vi "CPP_Aeroprobe.vi"() -> (5 "Plug in titles":string[](array[string]), 7 "Plug in values":string[](array[string]))   [LabVIEW 2022 SP3]
uses:
  Controls/AeroprobeType.ctl
  Controls/AeroprobeOrientation.ctl
  Plug in sub vis/CPP_Aeroprobe/eulerAngles.ctl
  <vilib>/Analysis/baseanly.llb/Mean (DBL).vi
  Globals/Meas_global.vi
  Globals/Constants_global.vi
  <vilib>/Utility/file.llb/Write Delimited Spreadsheet (DBL).vi
  <vilib>/Analysis/NI_AALBase.lvlib
panel:
  in  "manualOverride":bool
  in  "suppressNoiseWarning":bool
  out "PSU Warning":string
  in  "Probe:Euler:Angles":T1={"Roll"=-90.0, "Dip"=30.0, "Yaw"=0.0}
  out "Av Sampling Rate":dbl
  in  "Omniprobe Orientation":T2="30dip-EdgeTx {-90,30,0}"
  in  "Probe Type":T3=12 items=["5-Hole Probe"=5, "OmniProbe"=12]
  out "AeroFlow Output":cluster{string, string}[](array[cluster]) caption="Plug In Titles                                   Plug In Values"
  out "ZeroMeans&Vars":dbl[](array[numeric])
  in  "SaveTimeSeries?":bool
  in  "Mode":enum32{"Measure", "Take Zeroes"}(radio)
  in  "RunManually?":bool
  in  "MeanOrFull":bool
  in  "Graphs":bool
  in  "Downsampler":i32=40
  in  "Calibration Folder Path":path
  in  "Correction File Path":path
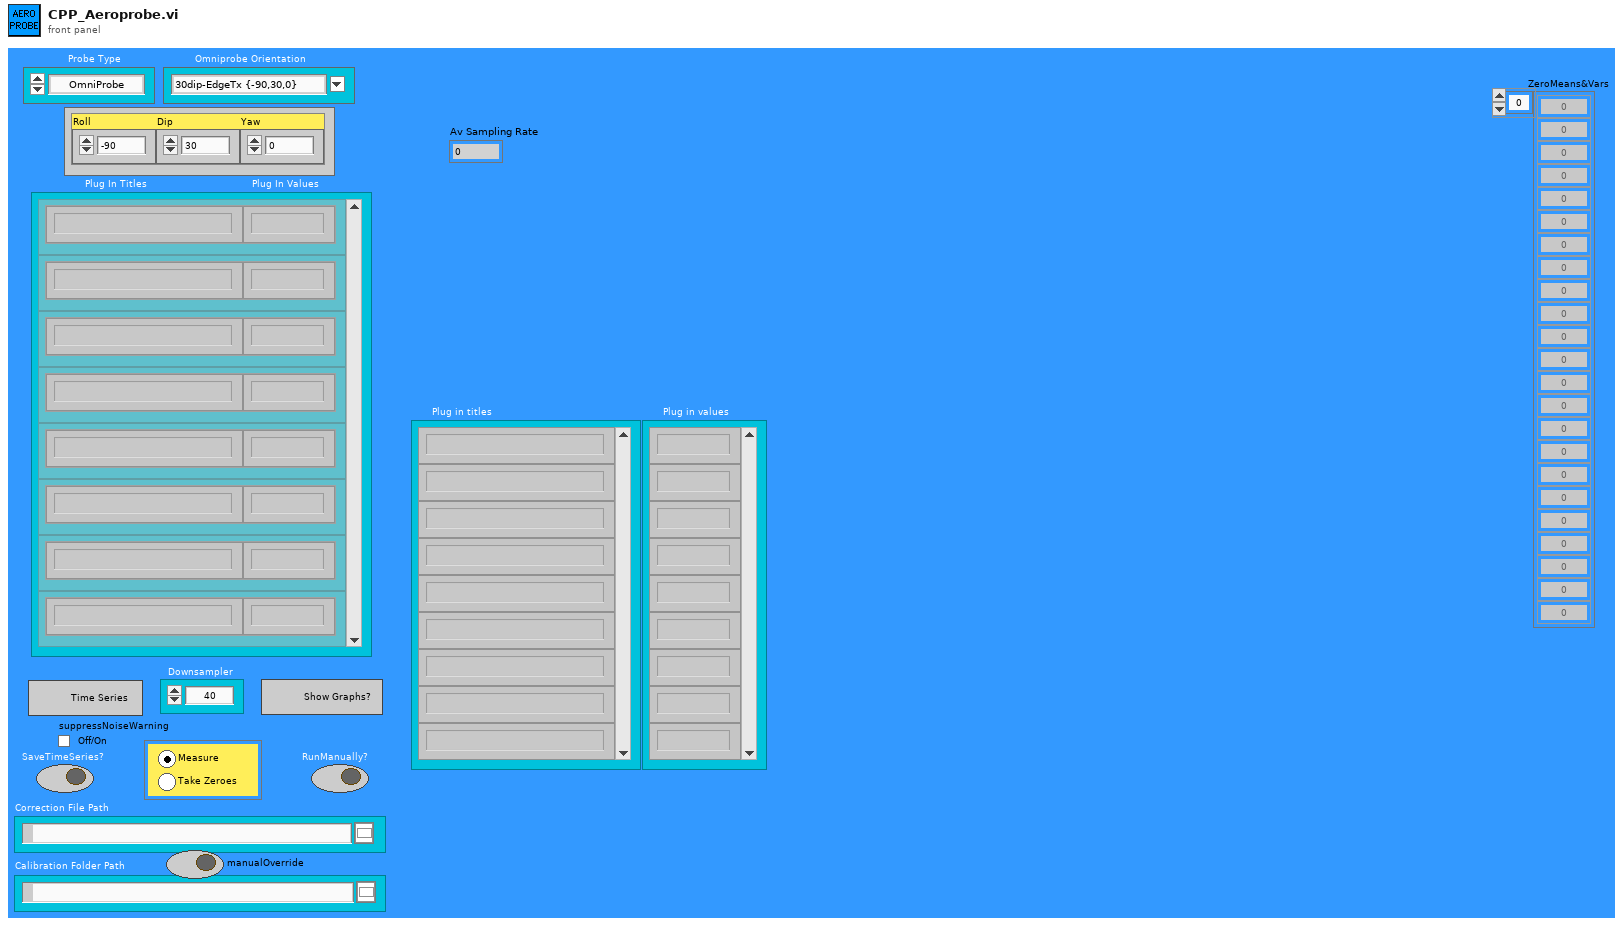
[diagram p1: front panel]
types:
  T1 = typedef "eulerAngles.ctl" = cluster{"Roll":dbl, "Dip":dbl, "Yaw":dbl}
  T2 = typedef "AeroprobeOrientation.ctl" = string
  T3 = typedef "AeroprobeType.ctl" = u16
  T4 = typedef "Post_Process.ctl" = enum16{"Take New Data", "Post Process Raw Data File"}
  T5 = enum16{"Raw Ends", "Mean Ends", "NaNd Ends", "Zeroed Ends"}
  T6 = enum16{"Save no data", "Save data in new files", "Save data in existing files"}
  T7 = typedef "Analysis_info_cluster.ctl" = cluster{"Colour":u32, "Inst type":T8, "Inst name":string, "Symbol":string, "Code name":string, "Extra Info":string, "Inst Array":T9, "Extra Titles":string[], "Extra Values":string[], "U":dbl, "u^2":dbl, "u^3":dbl, "u^4":dbl, "Skew_u":dbl, "Kurt_u":dbl, "Sd Error in Mean":dbl, "% u'/U":dbl, "X":dbl, "Y":dbl, "Z":dbl, "Timescale integral Estimate":dbl, "Sd Error in Variance":dbl, "Calib File":path, "Calib Constants":dbl[], "Output Position":bool, "Stats":enum16{"None", "Basic", "Full"}, "Av Sampling Rate":dbl, "Av No of Samples":dbl, "Total Meas Time (s)":dbl, "ADAM Ch Name":string, "Max value":dbl, "Min value":dbl, "Req Sample Rate Hz":dbl, "Sync Delay Time (s)":dbl, "Ch No":i16, "Device":string, "Use Latest Calib":bool, "Port":string, "Metadata Ch Names":string[], "Metadata Ch Values":string[], "Label":string}
  T8 = typedef "Inst_type.ctl" = enum16{"Raw voltage", "Raw with zero offsetting", "Propeller anemometer", "Pressure Transducer", "Pitot-static tube", "Hot wire", "Cross wire 1", "Cross wire 2", "Generic Linear", "Generic Polynomial", "Generic BackPoly", "Fast FID", "Thermocouple", "Cold wire", "Pulsed Wire", "LDA Vel", "LDA Tran time", "LDA Arr time", "Microphone"}
  T9 = typedef "Instrument_Array.ctl" = enum16{"PWA", "LDA", "Analogue"}
  T10 = typedef "Time_Trace_Cluster.ctl" = cluster{"Weighting":dbl[], "Voltage":dbl[], "Eng Values":dbl[]}
  T11 = cluster{"CleanVmagUVWCone":dbl[][], "CleanXvals":i32[]}
  T12 = typedef "SanityCluster.ctl" = cluster{"PressureErrors":bool[][], "Plug in titles":string[]}
  T13 = cluster{"   Vmag          U               V              W        Cone":dbl[][], "Xvals":i32[]}
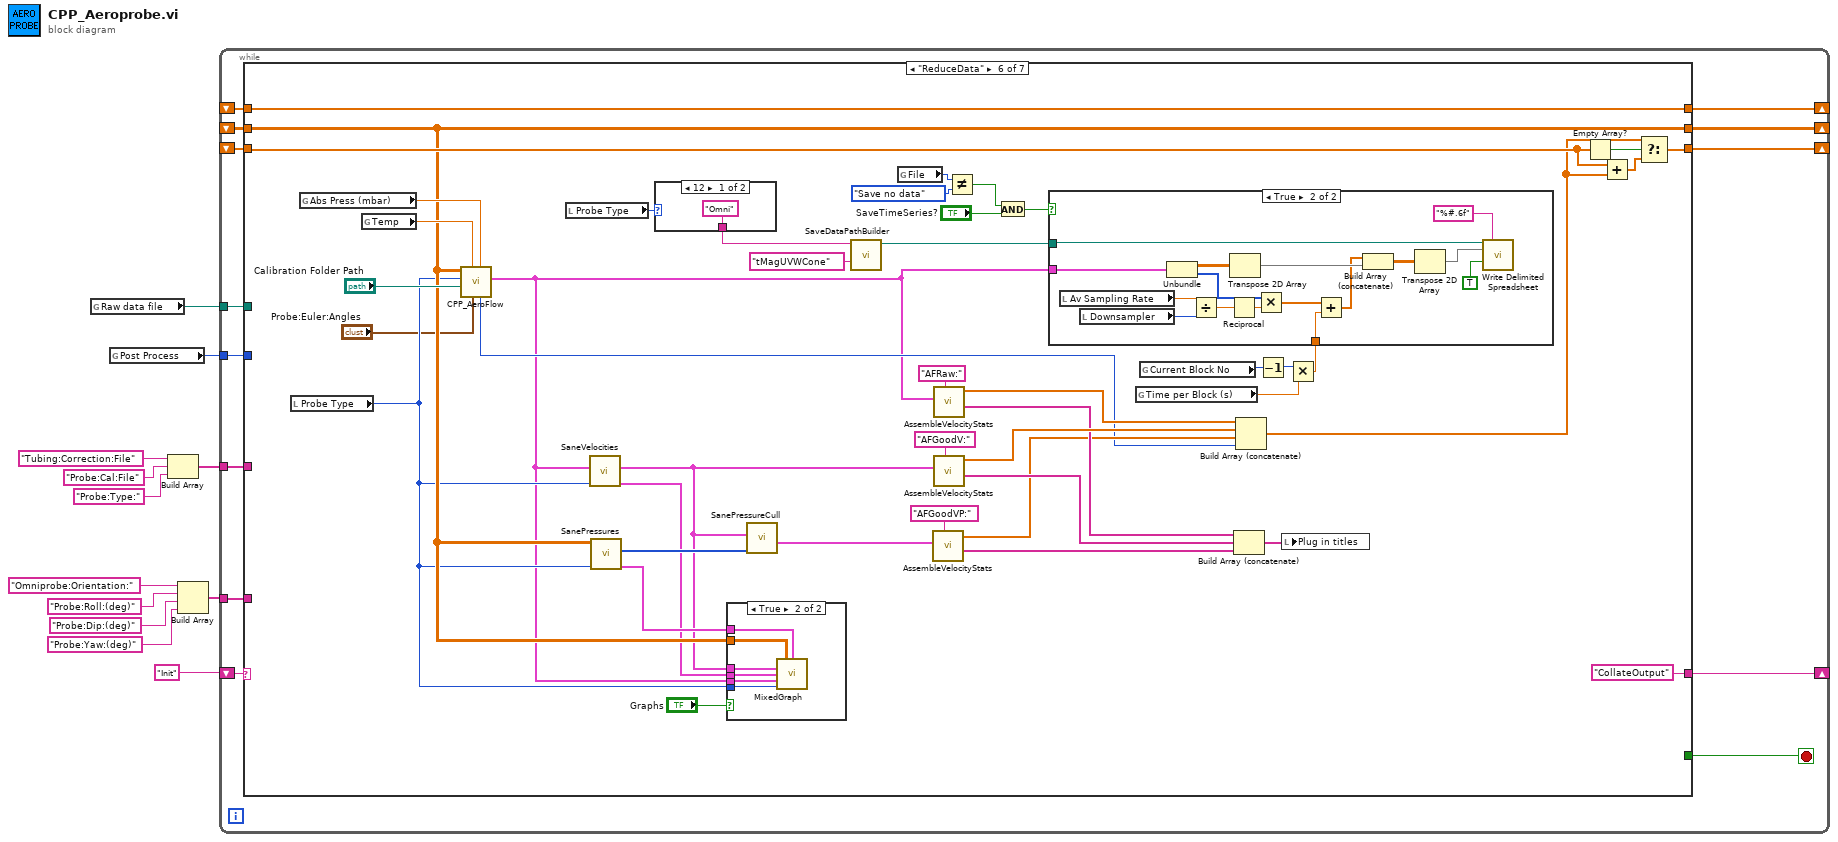
[diagram p0: block diagram]
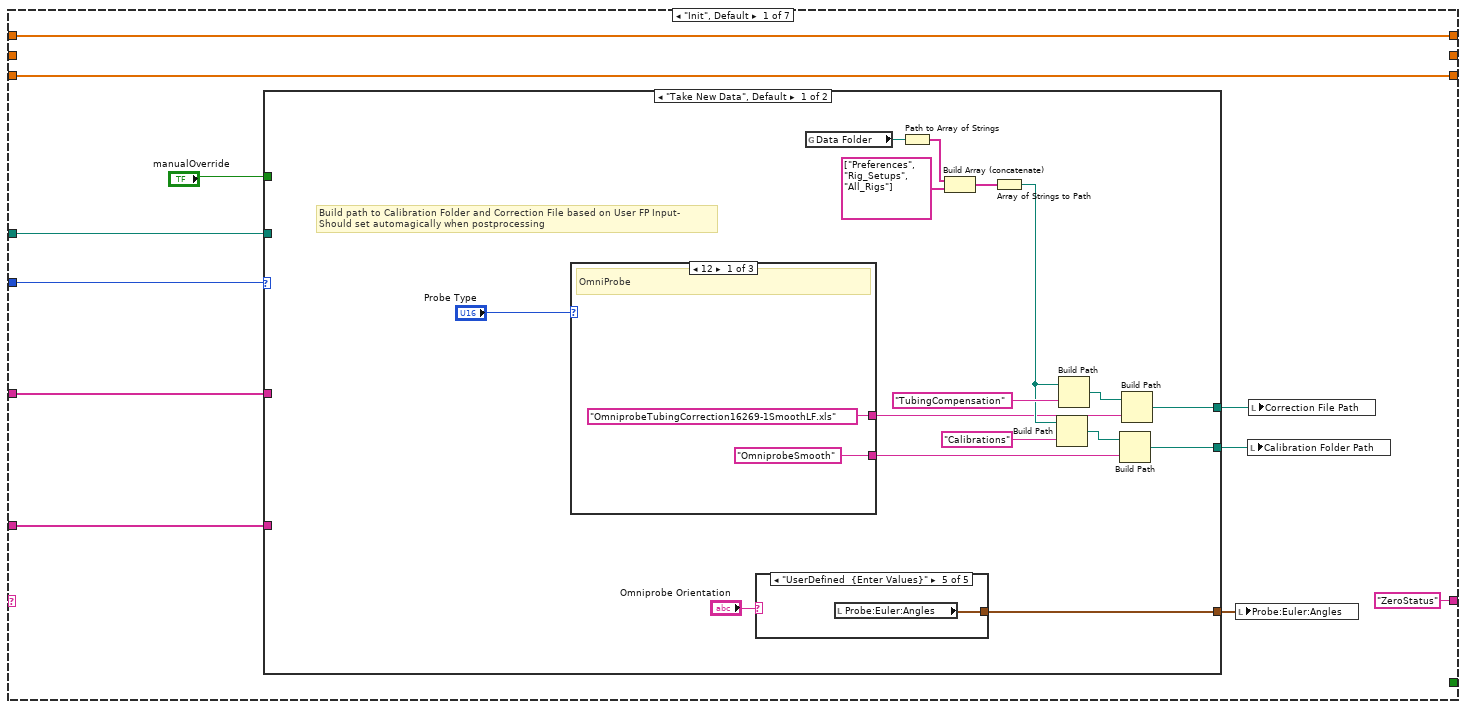
[diagram p2: hidden frame]
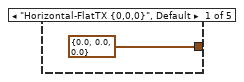
[diagram p3: hidden frame]
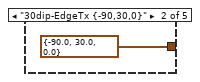
[diagram p4: hidden frame]
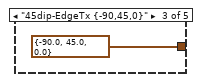
[diagram p5: hidden frame]
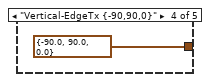
[diagram p6: hidden frame]
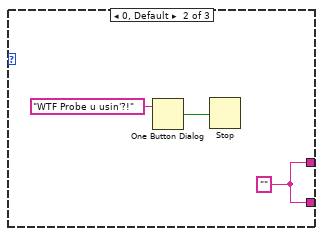
[diagram p7: hidden frame]
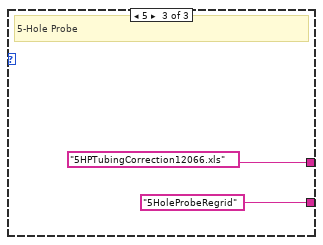
[diagram p8: hidden frame]
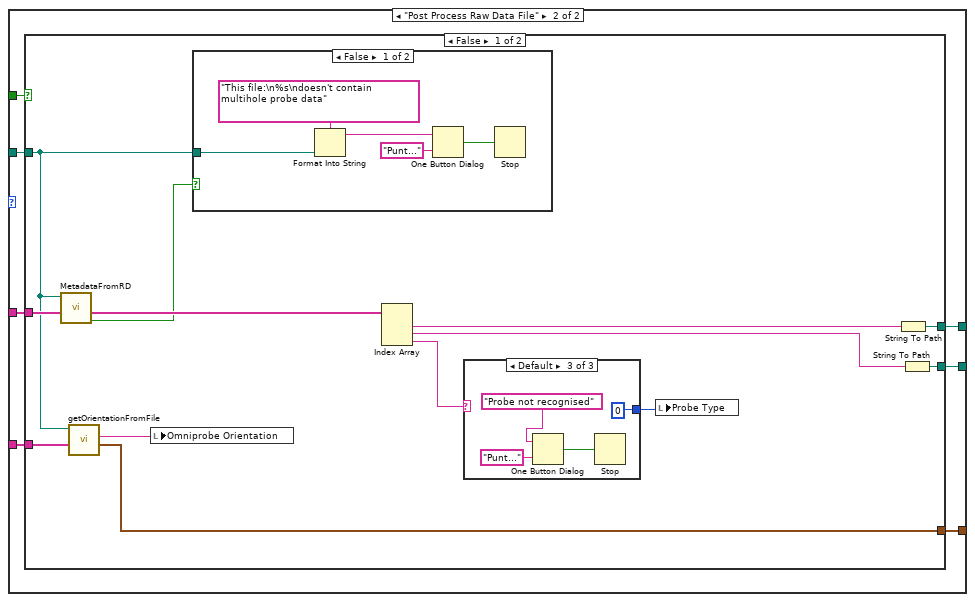
[diagram p9: hidden frame]
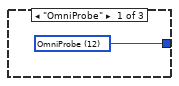
[diagram p10: hidden frame]
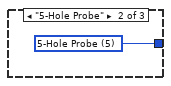
[diagram p11: hidden frame]
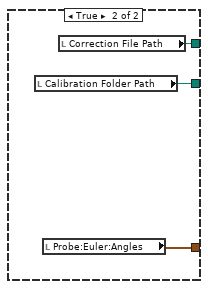
[diagram p13: hidden frame]
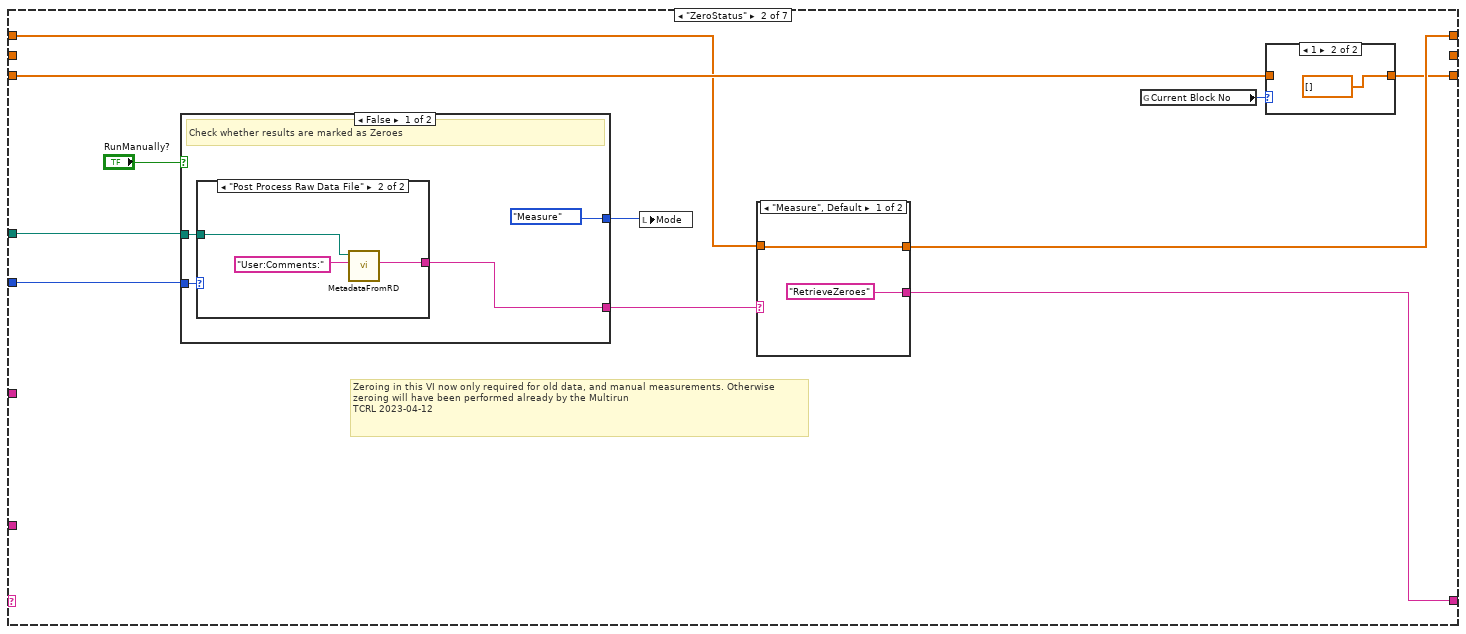
[diagram p14: hidden frame]
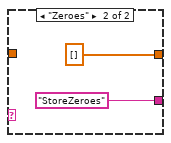
[diagram p15: hidden frame]
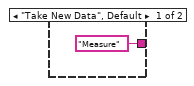
[diagram p16: hidden frame]
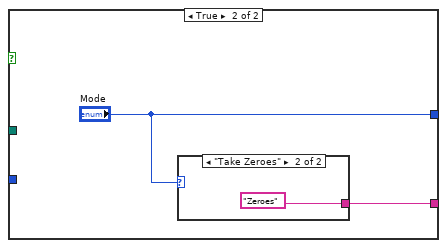
[diagram p17: hidden frame]
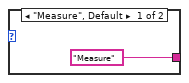
[diagram p18: hidden frame]
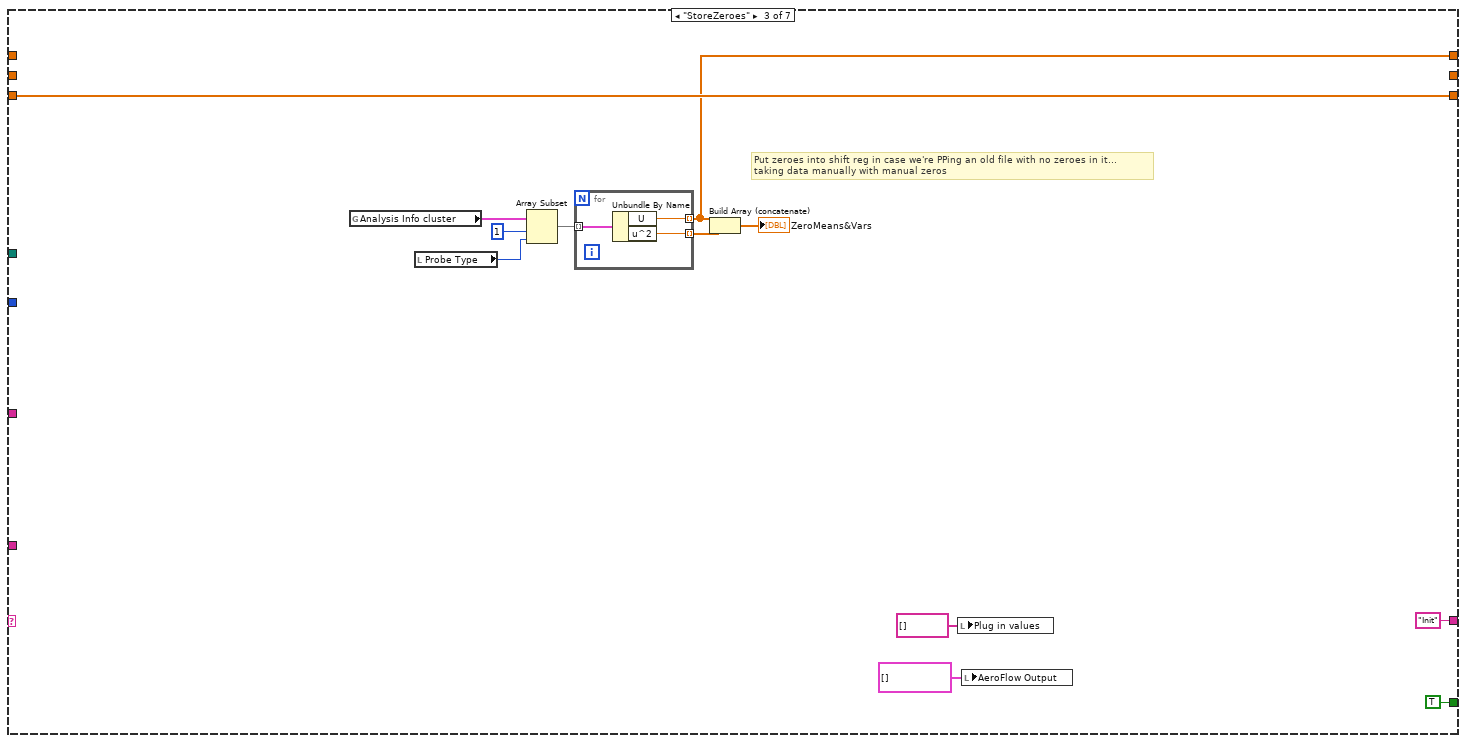
[diagram p20: hidden frame]
diagram:
  n1 = global read "Meas_global.vi" "Raw data file"() -> (w1:path)
  n2 = global read "Meas_global.vi" "Post Process"() -> (w11:T4)
  n3 = Build Array("Tubing:Correction:File" ("element"), "Probe:Cal:File" ("element"), "Probe:Type:" ("element")) -> (w4:string[])
  n4 = Build Array("Omniprobe:Orientation:" ("element"), "Probe:Roll:(deg)" ("element"), "Probe:Dip:(deg)" ("element"), "Probe:Yaw:(deg)" ("element")) -> (w6:string[])
  n5 = while {
    shift-right: [w24] -> _
    shift-left: "Init" -> [w25]
    shift-right: [w23] -> _
    shift-left: _ -> [w22]
    shift-right: [w21] -> _
    shift-left: _ -> [w20]
    shift-right: [w18] -> _
    shift-left: _ -> [w17]
    tunnel: w11 -> [w16]
    tunnel: w6 -> [w15]
    tunnel: w4 -> [w14]
    tunnel: w1 -> [w13]
    stop <- w19 stop-if-true
    n6 = case shown="\"ReduceData\"" w25 {
      tunnel: ["ZeroStatus" w101 "Init" w152 "ReduceData" "CollateOutput" "Init"] -> w24
      tunnel: [w36 w109 w133 w147 w191 w286 w348] -> w23
      tunnel: w22 -> [w36 w102 _ w149 w191 w286 w348]
      tunnel: [w35 w108 w139 w155 w193 w282 w342] -> w21
      tunnel: w20 -> [w35 w107 w139 w155 w193 w285 w342]
      tunnel: [_ _ TRUE w151 FALSE _ TRUE] -> w19
      tunnel: [_ _ _ w154 w188 w258 w344] -> w18
      tunnel: w17 -> [_ _ _ w154 _ w258 w344]
      tunnel: w16 -> [w31 w100 _ _ _ _ _]
      tunnel: w15 -> [w28 _ _ _ _ _ w314]
      tunnel: w14 -> [w30 _ _ _ _ _ w312]
      tunnel: w13 -> [w29 w99 _ w143 _ _ _]
      frame "Init", Default {
        n7 = case shown="\"Take New Data\", Default" w31 {
          tunnel: [w41 w69] -> w33
          tunnel: [w40 w70] -> w32
          tunnel: w30 -> [_ w71]
          tunnel: w29 -> [_ w68]
          tunnel: w28 -> [_ w67]
          tunnel: [w37 w66] -> w27
          tunnel: "manualOverride" -> [_ w65]
          frame "Take New Data", Default {
            # "Build path to Calibration Folder and Correction File based on User FP Input-\nShould set automagically when postprocessing"
            n8 = case shown="12" "Probe Type" {
              tunnel: ["OmniprobeTubingCorrection16269-1SmoothLF.xls" ("Tubing Compensation File") w62 "5HPTubingCorrection12066.xls" ("Tubing Compensation File")] -> w45
              tunnel: ["OmniprobeSmooth" ("Calibration Folder") w62 "5HoleProbeRegrid" ("Calibration Folder")] -> w44
              frame 12 {
                # "OmniProbe"
              }
              frame 0, Default {
                w62 = "" ("Calibration Folder")
                n9 = One Button Dialog(message="WTF Probe u usin'?!") -> (true=w60:bool)  [unwired: 1 in]
                n10 = Stop(stop? (T)=w60) -> ()
              }
              frame 5 {
                # "5-Hole Probe"
              }
            }
            n11 = case shown="\"UserDefined  {Enter Values}\"" "Omniprobe Orientation" {
              tunnel: [T1 {"Roll"=0.0, "Dip"=0.0, "Yaw"=0.0} ("Probe:Euler:Angles") T1 {"Roll"=-90.0, "Dip"=30.0, "Yaw"=0.0} ("Probe:Euler:Angles") T1 {"Roll"=-90.0, "Dip"=45.0, "Yaw"=0.0} ("Probe:Euler:Angles") T1 {"Roll"=-90.0, "Dip"=90.0, "Yaw"=0.0} ("Probe:Euler:Angles") w57] -> w37
              frame "Horizontal-FlatTX {0,0,0}", Default {
              }
              frame "30dip-EdgeTx {-90,30,0}" {
              }
              frame "45dip-EdgeTx {-90,45,0}" {
              }
              frame "Vertical-EdgeTx {-90,90,0}" {
              }
              frame "UserDefined  {Enter Values}" {
                n12 = local read "Probe:Euler:Angles"() -> (w57:T1)
              }
            }
            n13 = global read "Constants_global.vi" "Data Folder"() -> (w49:path)
            n14 = Path to Array of Strings(0:w49) -> (2:w52:string[])  [unwired: 1 out]
            n15 = Build Array (concatenate)(w52, string[] ["Preferences", "Rig_Setups", "All_Rigs"] ("array of strings 3")) -> (w50:string[])
            n16 = Array of Strings to Path(0:w50) -> (2:w46:path)  [unwired: 1 in]
            n17 = Build Path(base path=w46, name or relative path="Calibrations") -> (appended path=w42:path)
            n18 = Build Path(base path=w46, name or relative path="TubingCompensation") -> (appended path=w43:path)
            n19 = Build Path(base path=w42, name or relative path=w44) -> (appended path=w41:path)
            n20 = Build Path(base path=w43, name or relative path=w45) -> (appended path=w40:path)
          }
          frame "Post Process Raw Data File" {
            n21 = case shown="False" w65 {
              tunnel: w71 -> [w84 _]
              tunnel: [w81 w98] -> w70
              tunnel: [w79 w97] -> w69
              tunnel: w68 -> [w76 _]
              tunnel: w67 -> [w75 _]
              tunnel: [w74 w96] -> w66
              frame False {
                n22 = call "MetadataFromRD.vi"("ChannelNames"=w84, "Raw data file"=w76) -> ("allFound"=w78:bool, "ValueStrings"=w83:string[])  [unwired: 6 in, 2 out]
                n23 = call "getOrientationFromFile.vi"("currentChannels"=w75, "Raw data file"=w76) -> ("Probe:Euler:Angles"=w74:T1, "Omniprobe:Orientation"=w77:string)  [unwired: 8 in]
                n24 = local write "Omniprobe Orientation"(w77) -> ()
                n25 = case shown="False" w78 {
                  tunnel: w76 -> [w91 _]
                  frame False {
                    n26 = Format Into String(format string="This file:\n%s\ndoesn't contain multihole probe data" ("message"), w91) -> (resulting string=w94:string)  [unwired: 2 in, 1 out]
                    n27 = One Button Dialog(message=w94, button name ("OK")="Punt...") -> (true=w95:bool)
                    n28 = Stop(stop? (T)=w95) -> ()
                  }
                  frame True {
                  }
                }
                n29 = Index Array(array=w83) -> (element #1=w82:string, element #2=w80:string, element #3=w73:string)  [unwired: 3 in]
                n30 = case shown="Default" w73 {
                  tunnel: [w85 w86 0] -> w72
                  frame "OmniProbe" {
                    w85 = T3 12 items=["5-Hole Probe"=5, "OmniProbe"=12] ("Probe Type")
                  }
                  frame "5-Hole Probe" {
                    w86 = T3 5 items=["5-Hole Probe"=5, "OmniProbe"=12] ("Probe Type")
                  }
                  frame Default {
                    n31 = One Button Dialog(message="Probe not recognised", button name ("OK")="Punt...") -> (true=w89:bool)
                    n32 = Stop(stop? (T)=w89) -> ()
                  }
                }
                n33 = local write "Probe Type"(w72) -> ()
                n34 = String To Path(string=w82) -> (path=w81:path)
                n35 = String To Path(string=w80) -> (path=w79:path)
              }
              frame True {
                n36 = local read "Calibration Folder Path"() -> (w97:path)
                n37 = local read "Probe:Euler:Angles"() -> (w96:T1)
                n38 = local read "Correction File Path"() -> (w98:path)
              }
            }
          }
        }
        n39 = local write "Probe:Euler:Angles"(w27) -> ()
        n40 = local write "Calibration Folder Path"(w33) -> ()
        n41 = local write "Correction File Path"(w32) -> ()
      }
      frame "ZeroStatus" {
        # "Zeroing in this VI now only required for old data, and manual measurements. Otherwise zeroing will have been performed already by the Multirun\nTCRL 2023-04-12"
        n42 = case shown="False" "RunManually?" {
          tunnel: [enum32{"Measure", "Take Zeroes"}."Measure" ("Mode") "Mode"] -> w104
          tunnel: w100 -> [w117 _]
          tunnel: [w115 w122] -> w103
          tunnel: w99 -> [w114 _]
          frame False {
            # "Check whether results are marked as Zeroes"
            n43 = case shown="\"Post Process Raw Data File\"" w117 {
              tunnel: ["Measure" ("ValueString") w120] -> w115
              tunnel: w114 -> [_ w119]
              frame "Take New Data", Default {
              }
              frame "Post Process Raw Data File" {
                n44 = call "MetadataFromRD.vi"("ChannelName"="User:Comments:", "Raw data file"=w119) -> ("ValueString"=w120:string)  [unwired: 6 in, 3 out]
              }
            }
          }
          frame True {
            n45 = case shown="\"Take Zeroes\"" "Mode" {
              tunnel: ["Measure" ("y") "Zeroes" ("y")] -> w122
              frame "Measure", Default {
              }
              frame "Take Zeroes" {
              }
            }
          }
        }
        n46 = local write "Mode"(w104) -> ()
        n47 = case shown="\"Measure\", Default" w103 {
          tunnel: [w111 dbl[] [] ("t")] -> w109
          tunnel: w102 -> [w111 _]
          tunnel: ["RetrieveZeroes" "StoreZeroes"] -> w101
          frame "Measure", Default {
          }
          frame "Zeroes" {
          }
        }
        n48 = global read "Meas_global.vi" "Current Block No"() -> (w106:i32)
        n49 = case shown="1" w106 {
          tunnel: [w126 dbl[] [] ("t")] -> w108
          tunnel: w107 -> [w126 _]
          frame 0, Default {
          }
          frame 1 {
          }
        }
      }
      frame "StoreZeroes" {
        # "Put zeroes into shift reg in case we're PPing an old file with no zeroes in it...\ntaking data manually with manual zeros"
        n50 = global read "Meas_global.vi" "Analysis Info cluster"() -> (w137:T7[])
        n51 = local read "Probe Type"() -> (w135:T3)
        n52 = Array Subset(array=w137, index=1, length=w135) -> (w136:T7[])
        n53 = for {
          tunnel: w136 -> [w142] mode=indexing
          tunnel: [w141] -> w133 mode=indexing
          tunnel: [w140] -> w134 mode=indexing
          n54 = Unbundle By Name(w142) -> ("U"=w141:dbl, "u^2"=w140:dbl)
        }
        n55 = Build Array (concatenate)(w133, w134) -> (→"ZeroMeans&Vars":dbl[])
        n56 = local write "Plug in values"(string[] [] ("Plug in values")) -> ()
        n57 = local write "AeroFlow Output"(cluster{string, string}[] [] ("AeroFlow Output")) -> ()
      }
      frame "RetrieveZeroes" {
        # "Didn't find zeroes- hope they're in shift register"
        # "Found all the zeroes we need"
        # "Usual punt if we didn't get any zeroes\nNew data will either have been pre-zeroed by multirun, or manually zeroed in shift register\nIf we're postprocessing old data, zeros will be retrieved from RawDataFile"
        n58 = local read "Probe Type"() -> (w144:T3)
        n59 = call "findZerosInRD.vi"("Probe Type"=w144, "Raw data file"=w143) -> ("zerosChannels"=w145:string[])  [unwired: 9 in]
        n60 = call "RetrieveMetadataLiveOrPost.vi"("ChannelsToGet"=w145) -> ("ChannelValues"=w148:dbl[])  [unwired: 10 in]
        n61 = Add Array Elements(numeric array=w148) -> (sum=w153:dbl)
        n62 = Not A Number/Path/Refnum?(number/path/refnum=w153) -> (NaN/Path/Refnum?=w150:bool)
        n63 = Select(t=w149, s=w150, f=w148) -> (s? t:f=w147:dbl[])
        n64 = Empty Array?(array=w147) -> ()  [unwired: 1 out]
        n65 = case shown="False" FALSE {
          tunnel: ["CompensateData" "Init"] -> w152
          tunnel: [FALSE TRUE] -> w151
          frame False {
          }
          frame True {
            n66 = One Button Dialog(message="No zeroes. Try again.", button name ("OK")="OK") -> ()  [unwired: 1 out]
          }
        }
      }
      frame "CompensateData" {
        w186 = 1  # skip Pitot on Ch0
        # "Only subtract zeroes if there are some"
        # "Only complain if PSU in measurements"
        # "#Brittle\nTo cope with various Meas Setups"
        # "#FilthyHack"
        # "Using end-NaNd version of boosted data, to avoid the FFT' kicks that are frequently observed; hopefully AeroFlow can cope with NaNs..?!"
        n67 = global read "Meas_global.vi" "Analysis Info cluster"() -> (w169:T7[])
        n68 = local read "Probe Type"() -> (w179:T3)
        n69 = for {
          tunnel: w169 -> [w199] mode=indexing
          tunnel: [w198] -> w168
          tunnel: [w197] -> w167
          tunnel: [w194] -> w164
          tunnel: string[] ["Vsupply", "5V", "PSU"] -> [w196]
          stop <- w194 stop-if-true
          n70 = Unbundle By Name(w199) -> ("Inst name"=w195:string, "U"=w198:dbl, "u^2"=w197:dbl)
          n71 = for {
            tunnel: w196 -> [w203] mode=indexing
            tunnel: w195 -> [w201]
            tunnel: [w200] -> w194
            stop <- w200 stop-if-true
            n72 = Match Pattern(string=w201, regular expression=w203) -> (offset past match=w202:i32)  [unwired: 1 in, 3 out]
            n73 = Greater Or Equal To 0?(x=w202) -> (x >= 0?=w200:bool)
          }
        }
        n74 = global read "Meas_global.vi" "Time Trace"() -> (w180:T10[])
        n75 = case shown="12, Default" w179 {
          tunnel: [3e-07 ("y") 3.2e-07 ("y")] -> w177
          tunnel: [5e-08 ("y") 5e-08 ("y")] -> w178
          tunnel: [4.98 ("upper limit") 4.98 ("upper limit")] -> w176
          tunnel: [5.01 ("upper limit") 5.01 ("upper limit")] -> w175
          frame 5 {
          }
          frame 12, Default {
          }
        }
        n76 = Array Subset(array=w180, index=w186, length=w179) -> (w185:T10[])
        n77 = Index Array(array=w169, index=1) -> (element=w183:T7)
        n78 = Unbundle By Name(w183) -> ("Av Sampling Rate"=w181:dbl)
        "Av Sampling Rate" <- w181
        n79 = for {
          tunnel: w185 -> [w221] mode=indexing
          tunnel: [w220] -> w184 mode=indexing
          n80 = Unbundle By Name(w221) -> ("Eng Values"=w220:dbl[])
        }
        n81 = In Range and Coerce(upper limit=w175, x=w168, lower limit=w176) -> (In Range?=w174:bool)  [unwired: 1 out]
        n82 = In Range and Coerce(upper limit=w177, x=w167, lower limit=w178) -> (In Range?=w173:bool)  [unwired: 1 out]
        n83 = global read "Meas_global.vi" "Post Process"() -> (w172:T4)
        n84 = Compound Arithmetic op=OR(invert w174, invert w173) -> (w166:bool)
        n85 = Compound Arithmetic op=AND(w164, w166, invert "suppressNoiseWarning") -> (w165:bool)
        n86 = case shown="False" "MeanOrFull" {
          tunnel: [w226 w241] -> w192
          tunnel: w184 -> [w225 w240]
          tunnel: w181 -> [w222 _]
          frame False {
            # "Get the data off the global, and apply acoustic tubing correction. \nThen throw 90% of it away because we can't reduce it fast enough!"
            n87 = for {
              tunnel: w225 -> [w238] mode=indexing
              tunnel: [w235] -> w229 mode=indexing
              tunnel: TRUE ("Apply Phase Correction?") -> [w237]
              tunnel: "Correction File Path" -> [w236]
              tunnel: T5."NaNd Ends" ("EndTreatment") -> [w234]
              tunnel: 1.0 ("EndTrimLength(%)") -> [w233]
              tunnel: w222 -> [w232]
              workers-P: _ -> [_]
              n88 = call "GetCoeffsAndComp.vi"("EndTrimLength(%)"=w233, "EndTreatment"=w234, "Apply Phase Correction?"=w237, "Actual Sampling rate (Hz)"=w232, "mutedData"=w238, "TubingCorrectionFile"=w236) -> ("boostedData"=w235:dbl[])  [unwired: 5 in]
            }
            n89 = Transpose 2D Array(2D array=w229) -> (transposed array=w228:dbl[][])
            n90 = call "Decimator.vi"("Decimator"="Downsampler", "Array In"=w228) -> ("DecimatedArrayOut"=w226:dbl[][])  [unwired: 9 in]
          }
          frame True {
            # "Quick-and-dirty reduction of mean pressures"
            n91 = for {
              tunnel: w240 -> [w243] mode=indexing
              tunnel: [w242] -> w239 mode=indexing
              n92 = call-poly <vilib>:"Mean.vi"("X"=w243) -> ("mean"=w242:dbl)  [unwired: 1 out]
            }
            n93 = Build Array(w239) -> (w241:dbl[][])
          }
        }
        n94 = case shown="True" w165 {
          tunnel: w172 -> [_ w208]
          tunnel: ["" "Warning!\nAeroprobe PSU out of tolerance" ("PSU Warning")] -> w171
          tunnel: [FALSE ("Visible") TRUE ("Visible")] -> w170
          frame False {
          }
          frame True {
            # "Warn if 5V out of tolerance"
            n95 = case shown="\"Post Process Raw Data File\"" w208 {
              frame "Take New Data", Default {
                n96 = call "Email_With_Log.vi"("recipients"=string[] ["systems@cppwind.com"], "subject ([No Subject])"="Danger Will Robinson- OmniPSU", "message"="Warning! The Omniprobe 5V PSU is either off, or above its normal noise level- data will likely be junk!\n\nTry unplugging the Omniprobe PSU for 30s and plugging back in. Check with manual runs of Measurement that noise level is then acceptable.") -> ()  [unwired: 2 in, 2 out]
              }
              frame "Post Process Raw Data File" {
              }
            }
          }
        }
        "PSU Warning" <- w171
        n97 = call "SubtractZeroes.vi"("RawPressure"=w192, "Zeroes"=w191) -> ("ZeroedPressure"=w188:dbl[][])  [unwired: 9 in]
        n98 = property on="PSU Warning" class="Str"("Visible"=w170, "Blinking"=w170) -> ()  [unwired: 2 in, 2 out]
      }
      frame "ReduceData" {
        n99 = local read "Probe Type"() -> (w253:T3)
        n100 = global read "Meas_global.vi" "Abs Press (mbar)"() -> (w280:dbl)
        n101 = global read "Meas_global.vi" "Temp"() -> (w279:dbl)
        n102 = call "CPP_AeroFlow.vi"("Pressure (mBar)"=w280, "Probe:Euler:Angles"="Probe:Euler:Angles", "Temperature (C)"=w279, "Calibration Folder Path"="Calibration Folder Path", "Probe Type"=w253, "zeroedPress"=w258) -> ("Output"=w249:T11, "Time(ms)"=w257:u32)  [unwired: 2 in, 2 out]
        n103 = local read "Probe Type"() -> (w260:T3)
        n104 = call "SaneVelocities.vi"("Probe Type"=w253, "DataIn"=w249) -> ("VelocityErrors"=w252:T12, "DataOut"=w251:T13)  [unwired: 8 in]
        n105 = call "SanePressures.vi"("Probe Type"=w253, "ZeroedPressures"=w258) -> ("PressureIssues"=w256:T12, "XvalsGoodP"=w255:i32[])  [unwired: 8 in]
        n106 = case shown="12" w260 {
          tunnel: ["Omni" ("Inst name") "5HP" ("Inst name")] -> w259
          frame 12 {
          }
          frame 5, Default {
          }
        }
        n107 = case shown="True" "Graphs" {
          tunnel: w258 -> [_ w311]
          tunnel: w256 -> [_ w310]
          tunnel: w253 -> [_ w309]
          tunnel: w249 -> [_ w308]
          tunnel: w252 -> [_ w307]
          tunnel: w251 -> [_ w306]
          frame False {
          }
          frame True {
            n108 = call "MixedGraph.vi"("ZeroedPressures"=w311, "PressureSanity"=w310, "DataInClean"=w306, "CleaningErrors"=w307, "DataInRaw"=w308, "Probe Type"=w309) -> ()  [unwired: 10 in]
          }
        }
        n109 = call "SanePressureCull.vi"("GoodPressureXvals"=w255, "DataIn"=w251) -> ("DataOut"=w254:T13)  [unwired: 9 in]
        n110 = call "SaveDataPathBuilder.vi"("DataTypeSuffix"="tMagUVWCone", "Inst name"=w259) -> ("Path name Out"=w266:path)  [unwired: 9 in]
        n111 = global read "Meas_global.vi" "File"() -> (w264:T6)
        n112 = call "AssembleVelocityStats.vi"("TitlePrefix"="AFGoodVP:", "DataIn"=w254) -> ("Plug in titles"=w269:string[], "StatsArray"=w268:dbl[])  [unwired: 8 in]
        n113 = call "AssembleVelocityStats.vi"("TitlePrefix"="AFRaw:", "DataIn"=w249) -> ("Plug in titles"=w272:string[], "StatsArray"=w274:dbl[])  [unwired: 8 in]
        n114 = call "AssembleVelocityStats.vi"("TitlePrefix"="AFGoodV:", "DataIn"=w251) -> ("Plug in titles"=w271:string[], "StatsArray"=w273:dbl[])  [unwired: 8 in]
        n115 = Not Equal?(x=w264, y=T6."Save no data" ("File")) -> (x != y?=w261:bool)
        n116 = And(x=w261, y="SaveTimeSeries?") -> (x .and. y?=w262:bool)
        n117 = global read "Meas_global.vi" "Time per Block (s)"() -> (w246:dbl)
        n118 = global read "Meas_global.vi" "Current Block No"() -> (w248:i32)
        n119 = Build Array (concatenate)(w272, w271, w269) -> (w250:string[])
        n120 = Build Array (concatenate)(w274, w273, w268, w257) -> (w275:dbl[])
        n121 = Decrement(x=w248) -> (x-1=w247:i32)
        n122 = local write "Plug in titles"(w250) -> ()
        n123 = Multiply(x=w247, y=w246) -> (x*y=w245:dbl)
        n124 = case shown="True" w262 {
          tunnel: w266 -> [_ w305]
          tunnel: w249 -> [_ w297]
          tunnel: w245 -> [_ w291]
          frame False {
          }
          frame True {
            n125 = local read "Av Sampling Rate"() -> (w300:dbl)
            n126 = local read "Downsampler"() -> (w299:i32)
            n127 = Unbundle(w297) -> ("CleanVmagUVWCone"=w303:dbl[][], "CleanXvals"=w301:i32[])
            n128 = Divide(x=w300, y=w299) -> (x/y=w298:dbl)
            n129 = Reciprocal(x=w298) -> (1/x=w302:dbl)
            n130 = Transpose 2D Array(2D array=w303) -> (transposed array=w295:dbl[][])
            n131 = Multiply(x=w301, y=w302) -> (x*y=w294:dbl[])
            n132 = Add(x=w294, y=w291) -> (x+y=w292:dbl[])
            n133 = Build Array (concatenate)(w292, w295) -> (w296:dbl[][])
            n134 = Transpose 2D Array(2D array=w296) -> (transposed array=w293:dbl[][])
            n135 = call-poly <vilib>:"Write Delimited Spreadsheet.vi"("file path (dialog if empty)"=w305, "format (%.3f)"="%#.6f", "2D data"=w293, "append to file? (new file:F)"=TRUE) -> ()  [unwired: 10 in, 2 out]
          }
        }
        n136 = Empty Array?(array=w285) -> (empty?=w284:bool)
        n137 = Add(x=w285, y=w275) -> (x+y=w283:dbl[])
        n138 = Select(t=w275, s=w284, f=w283) -> (s? t:f=w282:dbl[])
      }
      frame "CollateOutput" {
        # "Calculate ensemble average"
        n139 = property on="Probe Type" class="Ring (strict)"() -> ("RingText.Text"=w327:string, "Value"=w317:T3)  [unwired: 2 in, 2 out]
        n140 = global read "Meas_global.vi" "Current Block No"() -> (w345:i32)
        n141 = case shown="12" w317 {
          tunnel: [w350 w362] -> w326
          tunnel: [w350 w361] -> w318
          tunnel: [w350 w353] -> w316
          tunnel: [w350 w352] -> w315
          tunnel: [string[] [] w351] -> w313
          tunnel: w314 -> [_ w351]
          frame 5, Default {
            w350 = ""
            # "5HP only to be used in regular vertical orientation; don't record orientation data."
          }
          frame 12 {
            n142 = local read "Probe:Euler:Angles"() -> (w360:T1)
            n143 = Unbundle By Name(w360) -> ("Roll"=w356:dbl, "Dip"=w355:dbl, "Yaw"=w354:dbl)
            n144 = Number To Fractional String(number=w356, precision (6)=i16 2) -> (F-format string=w361:string)  [unwired: 2 in]
            n145 = Number To Fractional String(number=w355, precision (6)=i16 2) -> (F-format string=w353:string)  [unwired: 2 in]
            n146 = Number To Fractional String(number=w354, precision (6)=i16 2) -> (F-format string=w352:string)  [unwired: 2 in]
            n147 = property on="Omniprobe Orientation" class="CmbBox (strict)"() -> ("Value"=w362:T2)  [unwired: 2 in, 2 out]
          }
        }
        n148 = local read "Downsampler"() -> (w341:i32)
        n149 = local read "MeanOrFull"() -> (w340:bool)
        n150 = local read "Calibration Folder Path"() -> (w330:path)
        n151 = local read "Correction File Path"() -> (w332:path)
        n152 = Divide(x=w342, y=w345) -> (x/y=w343:dbl[])
        n153 = Get Date/Time In Seconds() -> (seconds since 1Jan1904=w337:timestamp)
        n154 = Number To Decimal String(number=w341) -> (decimal integer string=w339:string)  [unwired: 1 in]
        n155 = To Double Precision Float(number=w337) -> (double precision float=w336:dbl)
        n156 = Number To Fractional String(number=w343) -> (F-format string=w333:string[])  [unwired: 3 in]
        n157 = Select(t="0", s=w340, f=w339) -> (s? t:f=w335:string)
        n158 = Path To String(path=w332) -> (string=w331:string)
        n159 = Number To Fractional String(number=w336, precision (6)=i16 3) -> (F-format string=w334:string)  [unwired: 2 in]
        n160 = Path To String(path=w330) -> (string=w329:string)
        n161 = Build Array (concatenate)(w333, w335, w334, w331, w329, w327, w326, w318, w316, w315) -> (w325:T2[])
        "Plug in values" <- w325
        n162 = local read "Plug in titles"() -> (w320:string[])
        n163 = Build Array (concatenate)(w320, "AFReduction:Time:(ms)", "Decimation:n:(0 for means only)" ("element"), "Reduction:Timestamp:(ss1-1-1904)" ("element"), w312, w313) -> (w319:string[])
        "Plug in titles" <- w319
        n164 = for {
          tunnel: w325 -> [w366] mode=indexing
          tunnel: w319 -> [w367] mode=indexing
          tunnel: [w368] -> w324 mode=indexing if=w363
          n165 = Empty String/Path?(string/path=w367) -> (empty?=w364:bool)
          n166 = Empty String/Path?(string/path=w366) -> (empty?=w365:bool)
          n167 = Bundle("element"=w367, "Value"=w366) -> (w368:cluster{"element":string, "Value":T2})  [unwired: 1 in]
          n168 = Not Or(1:w365, 2:w364) -> (0:w363:bool)
        }
        "AeroFlow Output" <- w324
      }
    }
  }
